vi "Address Space Size.vi"(2 "Basecard Config Registers":refnum<class "7902R Basecard Config Registers.lvclass">) -> (6 "size":u32)   [LabVIEW 2019, in "7902R Basecard Config Registers.lvclass"]
uses:
  7902R Basecard Config Registers.lvclass
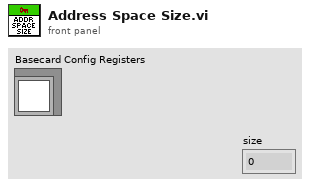
[diagram p1: front panel]
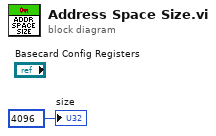
[diagram p0: block diagram]
diagram:
  "size" <- u32 4096 ("size")
